vi "Straight Edge Detection.vi"() -> ()   [LabVIEW 2014]
doc: "This example shows how to use Find Straight Edges in NI Vision. Find Straight Edges finds lines (or straight edges) within a search region. Find Straight Edges is a precursor function to many of the gauging and inspection tasks. For example, the location of the straight edges found within a region that encloses an object can interpreted as the boundaries of the object whose dimensions have to be measured for a gauging application or the presence of a crack in the surface of an object for an inspection application."
uses:
  <vilib>/vision/NI_Vision_Development_Module.lvlib
panel:
  out "Number of Lines Found":i32
  in  "Line Options":T1={"Number of Lines"=6, "Type"=4, "Minimum Score"=100.0, "Maximum Score"=1024.0, "Orientation"=0.0, "Angle Range"=10.0, "Angle Tolerance"=1.0, "Step Size"=3, "Min. SNR (db)"=0.0, "Min. Points (%)"=25.0, "Hough Iterations"=5} {"Min. Points (%)" min=0.0 max=100.0; "Min. SNR (db)" min=0.0; "Maximum Score" min=0.0 max=1024.0; "Minimum Score" min=1.0 max=1024.0 step=1.0; "Type" items=["First Edge Rake", "Best Edge Rake", "Hough Edge Rake", "First Edge Projection", "Best Edge Projection"]}
  in  "Edge Options":T2={"Edge Polarity"=0, "Kernel Size"=5, "Width"=3, "Minimum Edge Strength"=50.0, "Interpolation Type"=1, "Data Processing Method"=0} {"Data Processing Method" items=["Average", "Median"]; "Interpolation Type" items=["Zero Order"=0, "Bilinear"=1, "Bilinear Fixed"=4]; "Minimum Edge Strength" min=0.0 max=255.0 format="%.2g"; "Width" min=1 step=2; "Kernel Size" min=3 step=2; "Edge Polarity" items=["All Edges", "Rising Edges", "Falling Edges"]}
  in  "Search Direction":u32(ring) items=["Left to Right", "Right to Left", "Top to Bottom", "Bottom to Top"]
  out "Image":T3(plugin-control)
  in  "Stop":bool
  # "Overview: Demonstrates how to use the IMAQ Find Straight Edges function to find multiple straight lines in the Region of Interest (ROI).\nRequirements: Vision Development Software.\nInstructions: \n1. Run the VI.\n2. Draw a Region of Interest in the image, or modify the Edge Options or Line Options to see the straight edges the algorithm detects."
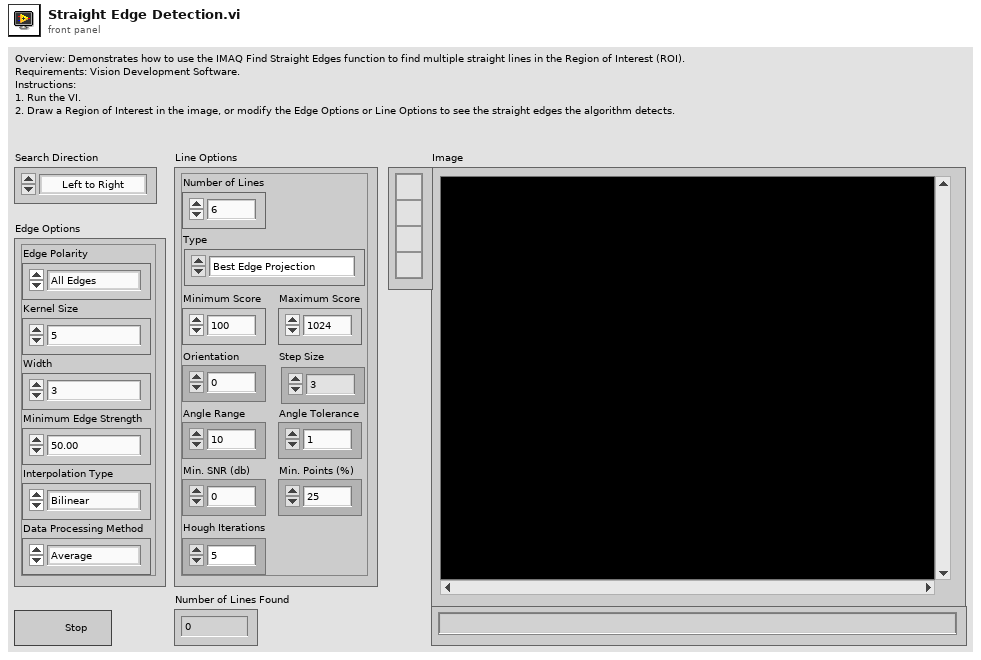
[diagram p1: front panel]
types:
  T1 = cluster{"Number of Lines":i32, "Type":u16, "Minimum Score":dbl, "Maximum Score":dbl, "Orientation":dbl, "Angle Range":dbl, "Angle Tolerance":dbl, "Step Size":u32, "Min. SNR (db)":dbl, "Min. Points (%)":dbl, "Hough Iterations":i32}
  T2 = cluster{"Edge Polarity":u16, "Kernel Size":u32, "Width":u32, "Minimum Edge Strength":dbl, "Interpolation Type":u16, "Data Processing Method":u16}
  T3 = typedef "IMAQ Image.ctl" = refnum<image>
  T4 = typedef "IMAQ Rectangle" = cluster{"Left":i32, "Top":i32, "Right":i32, "Bottom":i32, "Rotation":dbl}
  T5 = typedef "ROI Descriptor" = cluster{"Global Rectangle":i32[], "Contours":cluster{"ID":enum32{"External", "Internal"}, "Type":u32, "Coordinates":i32[]}[]}
  T6 = cluster{"Global Rectangle":i32[], "Contours":cluster{"Contour Type":u32, "ROI Type":u32, "Points":i32[]}[]}
  T7 = cluster{"Point1 (Pixels)":cluster{"X":sgl, "Y":sgl}, "Point2 (Pixels)":cluster{"X":sgl, "Y":sgl}, "Point1 (Real-World)":cluster{"X":sgl, "Y":sgl}, "Point2 (Real-World)":cluster{"X":sgl, "Y":sgl}, "Angle (Pixel)":dbl, "Angle (Real-World)":dbl, "Score":dbl, "Straightness":dbl, "Average SNR (db)":dbl, "Calibration Valid":bool}[]
  T8 = typedef "Search Line.ctl" = cluster{"Start Point":cluster{"X":sgl, "Y":sgl}, "End Point":cluster{"X":sgl, "Y":sgl}, "Edge Info":T9[], "Edge Map":dbl[], "Calibration Valid":bool}
  T9 = typedef "Edge New.ctl" = cluster{"Location (Pixel)":cluster{"X":sgl, "Y":sgl}, "Location (Real-World)":cluster{"X":sgl, "Y":sgl}, "Distance (Pixel)":dbl, "Distance (Real-World)":dbl, "Strength":dbl, "Noise":dbl, "Rising?":bool}
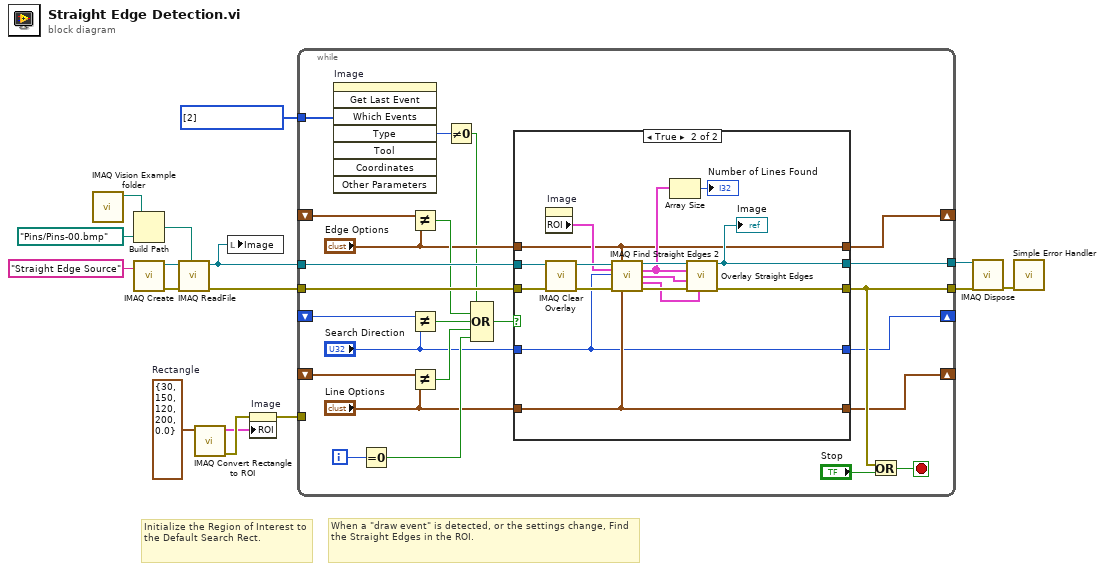
[diagram p0: block diagram]
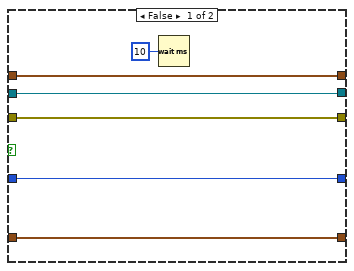
[diagram p2: hidden frame]
diagram:
  w4 = i32[] [2] items=["No Event"=0, "Click Event"=1, "Draw Event"=2, "Size Event"=4, "Scroll Event"=5, "Double Click Event"=8] ("Which Events")
  w5 = T4 {"Left"=30, "Top"=150, "Right"=120, "Bottom"=200, "Rotation"=0.0}  # Rectangle
  # "When a \"draw event\" is detected, or the settings change, Find the Straight Edges in the ROI."
  # "Initialize the Region of Interest to the Default Search Rect."
  n1 = call "IMAQ Vision Example folder.vi"() -> ("Example Image Path"=w11:path)  [unwired: 11 in]
  n2 = Build Path(base path=w11, name or relative path=path "Pins/Pins-00.bmp") -> (appended path=w14:path)
  n3 = call "IMAQ Create"("Image Name"="Straight Edge Source") -> ("New Image"=w10:T3, "error out"=w12:errorcluster)  [unwired: 4 in]
  n4 = call "IMAQ ReadFile"("File Path"=w14, "error in (no error)"=w12, "Image"=w10) -> ("error out"=w6:errorcluster, "Image Out"=w7:T3)  [unwired: 4 in, 3 out]
  n5 = call "IMAQ Convert Rectangle to ROI"("Rectangle"=w5) -> ("error out"=w3:errorcluster, "ROI Descriptor"=w2:T5)  [unwired: 8 in]
  n6 = local write "Image"(w7) -> ()
  n7 = property on="Image" class="ImageControl"(error in=w3, "ROI"=w2) -> (error out=w1:errorcluster)  [unwired: 1 in, 1 out]
  n8 = while {
    tunnel: w7 -> [w40]
    tunnel: [w24] -> w9
    tunnel: [w39] -> w8
    tunnel: w6 -> [w38]
    shift-right: [w17] -> _
    shift-left: _ -> [w35]
    shift-right: [w18] -> _
    shift-left: _ -> [w37]
    shift-right: [w19] -> _
    shift-left: _ -> [w36]
    tunnel: w4 -> [w22]
    tunnel: w1 -> [_]
    i -> [w34]
    stop <- w23 stop-if-true
    n9 = invoke on="Image" class="ImageControl" method="Get Last Event"("Which Events"=w22) -> ("Type"=w21:i32)  [unwired: 7 in, 7 out]
    n10 = Equal To 0?(x=w34) -> (x = 0?=w30:bool)
    n11 = Not Equal?(x=w35, y="Edge Options") -> (x != y?=w29:bool)
    n12 = Not Equal?(x=w37, y="Search Direction") -> (x != y?=w33:bool)
    n13 = Not Equal?(x=w36, y="Line Options") -> (x != y?=w31:bool)
    n14 = Not Equal To 0?(x=w21) -> (x != 0?=w20:bool)
    n15 = Compound Arithmetic op=OR(w20, w29, w33, w31, w30) -> (w32:bool)
    n16 = case shown="True" w32 {
      tunnel: w40 -> [w46 w62]
      tunnel: [w46 w61] -> w39
      tunnel: w38 -> [w45 w60]
      tunnel: [w45 w59] -> w24
      tunnel: "Edge Options" -> [w41 w47]
      tunnel: "Search Direction" -> [w43 w48]
      tunnel: "Line Options" -> [w44 w49]
      tunnel: [w44 w49] -> w19
      tunnel: [w43 w48] -> w18
      tunnel: [w41 w47] -> w17
      frame False {
        n17 = Wait (ms)(milliseconds to wait=u32 10) -> ()  [unwired: 1 out]
      }
      frame True {
        n18 = property on="Image" class="ImageControl"() -> ("ROI"=w56:T6)  [unwired: 2 in, 2 out]
        n19 = call "IMAQ Clear Overlay"("error in (no error)"=w60, "Image"=w62) -> ("error out"=w58:errorcluster, "Image Out"=w57:T3)  [unwired: 8 in]
        n20 = call "IMAQ Find Straight Edges 2"("Image"=w57, "Edge Options"=w47, "ROI Descriptor"=w56, "Search Direction"=w48, "error in (no error)"=w58, "Line Options"=w49) -> ("Image (duplicate)"=w55:T3, "Straight Edges"=w51:T7, "Search Lines Information"=w54:T8[], "Used Edges"=w52:cluster{"Edge Information":T9[]}[], "error out"=w53:errorcluster)  [unwired: 5 in]
        n21 = Array Size(array=w51) -> (size(s)=→"Number of Lines Found":i32)
        n22 = call "Overlay Straight Edges.vi"("All Edges (Pixel)"=w52, "error in"=w53, "Search Lines Information"=w54, "Straight Edges"=w51, "Image In"=w55) -> ("error out"=w59:errorcluster, "Image Out"=w61:T3)  [unwired: 5 in]
        "Image" <- w61
      }
    }
    n23 = Or(x=w24, y="Stop") -> (x .or. y?=w23:bool)
  }
  n24 = call "IMAQ Dispose"("Image"=w8, "error in (no error)"=w9) -> ("error out"=w16:errorcluster)  [unwired: 4 in]
  n25 = call <vilib>:"Simple Error Handler.vi"("error in (no error)"=w16) -> ()  [unwired: 4 in, 5 out]
